vi "worksheet filter column lv.vi"(8 "error in (no error)":errorcluster, 9 "lxw_filter_rule":T3 {"criteria" items=["LXW_FILTER_CRITERIA_NONE", "LXW_FILTER_CRITERIA_EQUAL_TO", "LXW_FILTER_CRITERIA_NOT_EQUAL_TO", "LXW_FILTER_CRITERIA_GREATER_THAN", "LXW_FILTER_CRITERIA_LESS_THAN", "LXW_FILTER_CRITERIA_GREATER_THAN_OR_EQUAL_TO", "LXW_FILTER_CRITERIA_LESS_THAN_OR_EQUAL_TO", "LXW_FILTER_CRITERIA_BLANKS", "LXW_FILTER_CRITERIA_NON_BLANKS"]}, 10 "col":u16, 11 "worksheet":u32) -> (0 "error out":errorcluster, 2 "rule":T2 {"criteria" items=["LXW_FILTER_CRITERIA_NONE", "LXW_FILTER_CRITERIA_EQUAL_TO", "LXW_FILTER_CRITERIA_NOT_EQUAL_TO", "LXW_FILTER_CRITERIA_GREATER_THAN", "LXW_FILTER_CRITERIA_LESS_THAN", "LXW_FILTER_CRITERIA_GREATER_THAN_OR_EQUAL_TO", "LXW_FILTER_CRITERIA_LESS_THAN_OR_EQUAL_TO", "LXW_FILTER_CRITERIA_BLANKS", "LXW_FILTER_CRITERIA_NON_BLANKS"]}, 3 "function return":u32(ring))   [LabVIEW 8.6]
doc: "lxw_error worksheet_filter_column(lxw_worksheet worksheet, lxw_col_t col, unsigned long rule);"
uses:
  pending_lvxlsxwriter/xlsxwriter.dll
  Controls/lxw_filter_criteria.ctl
  Controls/lxw_filter_rule.ctl
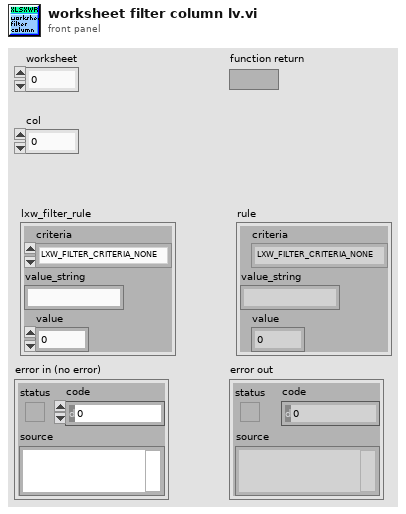
[diagram p1: front panel]
types:
  T1 = typedef "lxw_filter_criteria.ctl" = u32
  T2 = cluster{"criteria":T1, "value_string":string, "value":dbl}
  T3 = typedef "lxw_filter_rule.ctl" = cluster{"criteria":T1, "value_string":string, "value":dbl}
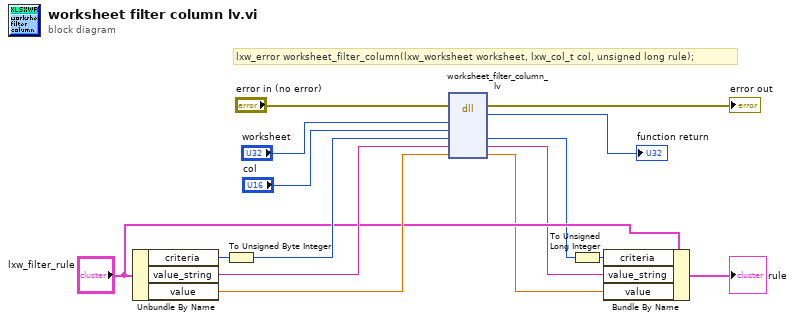
[diagram p0: block diagram]
diagram:
  # "lxw_error worksheet_filter_column(lxw_worksheet worksheet, lxw_col_t col, unsigned long rule);"
  n1 = Unbundle By Name("lxw_filter_rule") -> ("criteria"=w7:T1, "value_string"=w9:string, "value"=w8:dbl)
  n2 = To Unsigned Byte Integer(number=w7) -> (unsigned 8bit integer=w11:u8)
  n3 = dll-call lib="C:/Users/WDAGUtilityAccount/Desktop/pending_lvxlsxwriter/xlsxwriter.*" fn="worksheet_filter_column_lv"(error in="error in (no error)", "worksheet"="worksheet", "col"="col", "criteria"=w11, "value_string"=w9, "value"=w8) -> (error out=→"error out":errorcluster, "return type"=→"function return":u32, "criteria"=w4:u8, "value_string"=w3:string, "value"=w2:dbl)  [unwired: 4 in, 1 out]
  n4 = To Unsigned Long Integer(number=w4) -> (unsigned 32bit integer=w5:u32)
  n5 = Bundle By Name(cluster="lxw_filter_rule", "criteria"=w5, "value_string"=w3, "value"=w2) -> (→"rule":T3)
